vi "102_Lipgap_Full_Algo_new.vi"(0 "Image":T4(plugin-control), 1 "Calibrated Image":T4, 2 "Reference ROI":T5 {"Contours"."Type" items=["No Selection", "Point", "Line", "Rectangle", "Oval", "Polygon", "Freehand Region", "Annulus", "Unused2", "Unused3", "Broken Line", "Freehand Line", "Rotated Rectangle"]}, 3 "Line Options ROI Ref":T9={"Number of Lines"=1, "Type"=enum."First Edge Rake", "Min. Score"=10.0, "Max. Score"=1000.0, "Orientation"=0.0, "Angle Range"=45.0, "Angle Tolerance"=1.0, "Step Size"=3, "Min. SNR (db)"=0.0, "Min. Points (%)"=25.0, "Hough Iterations"=5} {"Min. Points (%)" min=0.0 max=100.0; "Min. SNR (db)" min=0.0; "Max. Score" min=0.0 max=1024.0; "Min. Score" min=0.0 max=1024.0 step=1.0}, 4 "Edge Options ROI Ref":T6={"Edge Polarity"=0, "Kernel Size"=3, "Width"=3, "Minimum Edge Strength"=50.0, "Interpolation Type"=enum."Zero Order", "Data Processing Method"=enum."Average"} {"Edge Polarity" items=["All Edges", "Rising Edges", "Falling Edges"]; "Minimum Edge Strength" format="%.2f"; "Width" step=2; "Kernel Size" step=2}, 5 "Search Direction ROI Ref":u32=3, 6 "Measurement ROI 1":T5 {"Contours"."Type" items=["No Selection", "Point", "Line", "Rectangle", "Oval", "Polygon", "Freehand Region", "Annulus", "Unused2", "Unused3", "Broken Line", "Freehand Line", "Rotated Rectangle"]}, 7 "error in (no error)":errorcluster, 8 "Blob Center":cluster{"Center X":dbl, "Center Y":dbl}, 9 "Search Direction ROI 1":u16(ring)=2 items=["Left To Right", "Right To Left", "Top To Bottom", "Bottom To Top"], 10 "Edge Options ROI 1":T6={"Edge Polarity"=0, "Kernel Size"=3, "Width"=3, "Minimum Edge Strength"=50.0, "Interpolation Type"=enum."Zero Order", "Data Processing Method"=enum."Average"} {"Edge Polarity" items=["All Edges", "Rising Edges", "Falling Edges"]; "Minimum Edge Strength" format="%.2f"; "Width" step=2; "Kernel Size" step=2}, 11 "Measurement ROI 2":T5 {"Contours"."Type" items=["No Selection", "Point", "Line", "Rectangle", "Oval", "Polygon", "Freehand Region", "Annulus", "Unused2", "Unused3", "Broken Line", "Freehand Line", "Rotated Rectangle"]}, 12 "Scan Direction ROI 2":u16(ring) items=["Left To Right", "Right To Left", "Top To Bottom", "Bottom To Top"], 13 "Edge Options ROI 2":T6={"Edge Polarity"=0, "Kernel Size"=3, "Width"=3, "Minimum Edge Strength"=10.0, "Interpolation Type"=enum."Bilinear Fixed", "Data Processing Method"=enum."Average"} {"Edge Polarity" items=["All Edges", "Rising Edges", "Falling Edges"]; "Minimum Edge Strength" format="%.2f"; "Width" step=2; "Kernel Size" step=2}, 14 "Process ROI 2":T8(ring)=enum."Get All Edges", 15 "Step Size ROI 2":u32=5) -> (18 "Overlay Arrow Lines":T1, 20 "Real World Lip Gap 102":sgl, 27 "error IO":errorcluster)   [LabVIEW 2019, in "Algorithm.lvclass"]
uses:
  FrameworkOverrides/Algorithm.lvclass
  <vilib>/vision/NI_Vision_Development_Module.lvlib
  <vilib>/vision/Measure.llb/Edge Polarity.ctl
  <vilib>/vision/Measure.llb/Edge Options.ctl
  <vilib>/vision/Measure.llb/Straight Edge Process.ctl
  <vilib>/vision/Measure.llb/Straight Edge Options.ctl
  <vilib>/vision/Image Controls.llb/IMAQ Image.ctl
panel:
  out "Second Overlay Line":T2
  out "First Overlay Line":T3
  out "Array":i32[](array[numeric])
  out "min value":sgl
  out "max value":sgl
  out "x/y":sgl
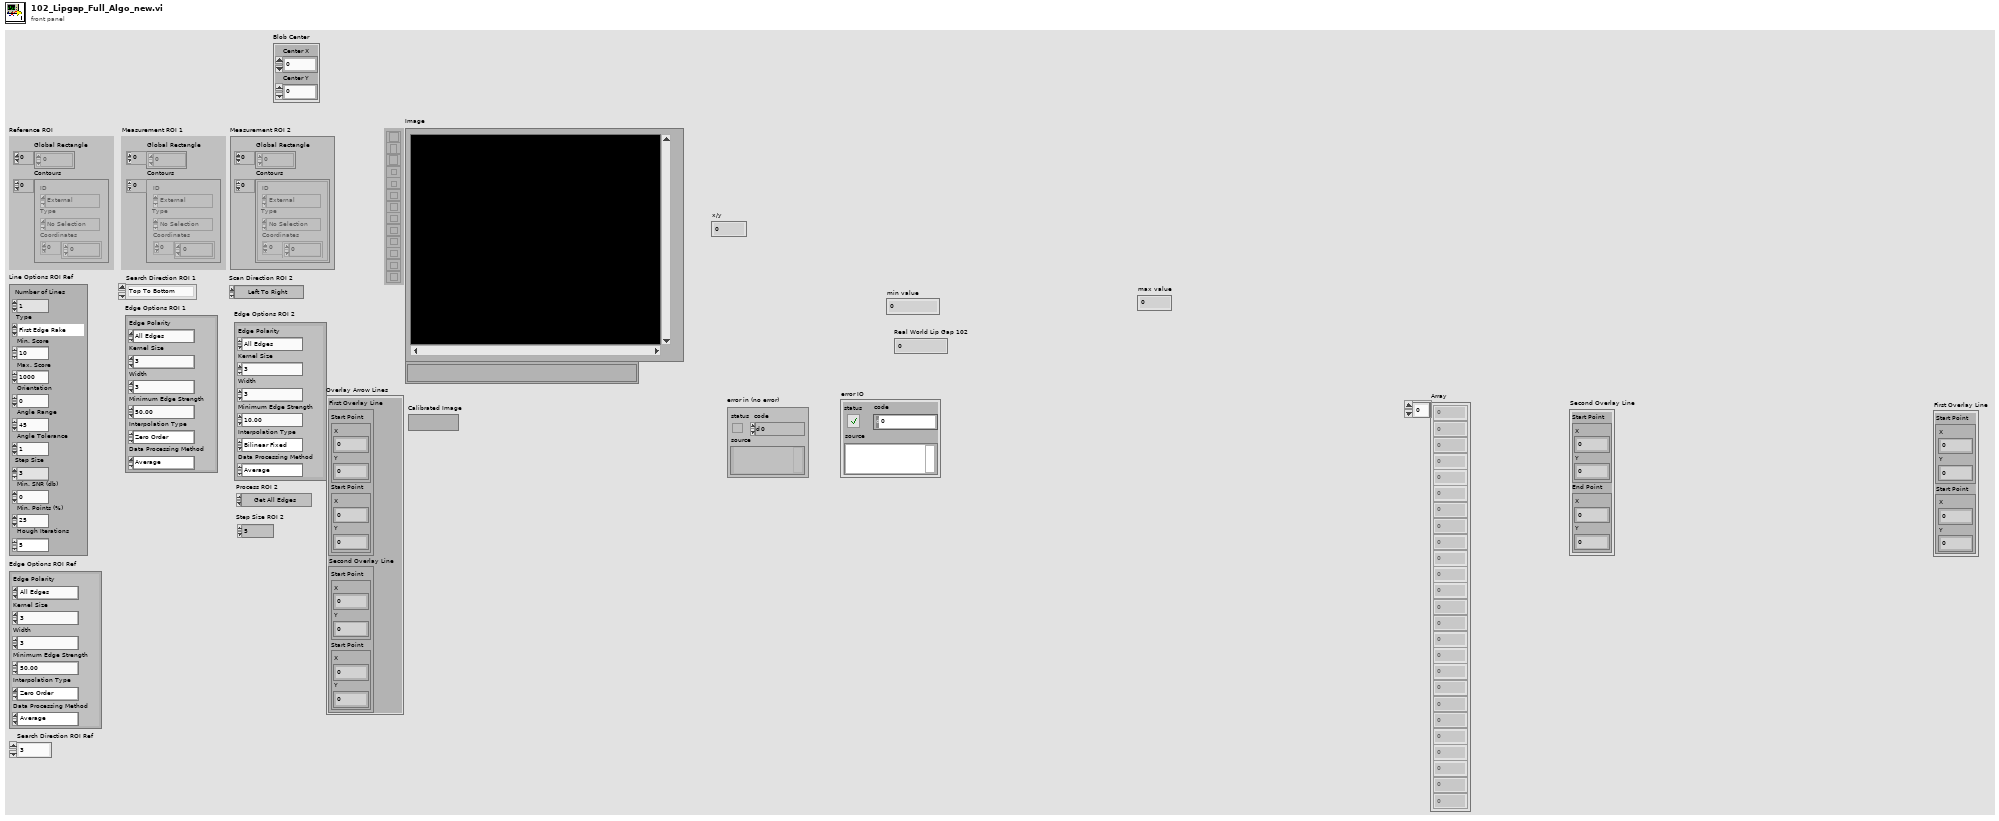
[diagram p1: front panel]
types:
  T1 = cluster{"First Overlay Line ":cluster{"Start Point":cluster{"X":sgl, "Y":sgl}, "Start Point":cluster{"X":sgl, "Y":sgl}}, "Second Overlay Line ":cluster{"Start Point":cluster{"X":sgl, "Y":sgl}, "Start Point":cluster{"X":sgl, "Y":sgl}}}
  T2 = cluster{"Start Point":cluster{"X":sgl, "Y":sgl}, "End Point":cluster{"X":sgl, "Y":sgl}}
  T3 = cluster{"Start Point":cluster{"X":sgl, "Y":sgl}, "Start Point":cluster{"X":sgl, "Y":sgl}}
  T4 = typedef "IMAQ Image.ctl" = refnum<image>
  T5 = typedef "ROI Descriptor" = cluster{"Global Rectangle":i32[], "Contours":cluster{"ID":enum32{"External", "Internal"}, "Type":u32, "Coordinates":i32[]}[]}
  T6 = typedef "Edge Options.ctl" = cluster{"Edge Polarity":T7, "Kernel Size":u32, "Width":u32, "Minimum Edge Strength":sgl, "Interpolation Type":enum32{"Zero Order", "Bilinear", "Quadratic", "Cubic", "Bilinear Fixed"}, "Data Processing Method":enum32{"Average", "Median"}}
  T7 = typedef "Edge Polarity.ctl" = u32
  T8 = enum16{"Get First Edge", "Get First + Last Edge", "Get All Edges", "Get Best Edge"}
  T9 = typedef "Straight Edge Options.ctl" = cluster{"Number of Lines":i32, "Type":T10, "Min. Score":dbl, "Max. Score":dbl, "Orientation":dbl, "Angle Range":dbl, "Angle Tolerance":dbl, "Step Size":u32, "Min. SNR (db)":dbl, "Min. Points (%)":dbl, "Hough Iterations":i32}
  T10 = typedef "Straight Edge Process.ctl" = enum32{"First Edge Rake", "Best Edge Rake", "Hough Edge Rake", "First Edge Projection", "Best Edge Projection"}
  T11 = typedef "IMAQ Rectangle" = cluster{"Left":i32, "Top":i32, "Right":i32, "Bottom":i32, "Rotation":dbl}
  T12 = cluster{"Left":dbl, "Top":dbl, "Right":dbl, "Bottom":dbl, "Angle":dbl}
  T13 = cluster{"Search Direction":u32, "Edge Options":T6, "Show Search Area":bool, "Show Search Lines":bool, "Show Edges Found":bool, "Show Result":bool, "Search Area Color":u32, "Search Lines Color":u32, "Edge Locations Color":u32, "Result Color":u32, "Overlay Group Name":string}
  T14 = cluster{"Point1 (Pixels)":cluster{"X":sgl, "Y":sgl}, "Point2 (Pixels)":cluster{"X":sgl, "Y":sgl}, "Point1 (Real-World)":cluster{"X":sgl, "Y":sgl}, "Point2 (Real-World)":cluster{"X":sgl, "Y":sgl}, "Angle (Pixel)":dbl, "Angle (Real-World)":dbl, "Score":dbl, "Straightness":dbl, "Average SNR (db)":dbl, "Calibration Valid":bool}[]
  T15 = cluster{"Point1 (Pixels)":cluster{"X":sgl, "Y":sgl}, "Point2 (Pixels)":cluster{"X":sgl, "Y":sgl}, "Point1 (Real-World)":cluster{"X":sgl, "Y":sgl}, "Point2 (Real-World)":cluster{"X":sgl, "Y":sgl}, "Angle (Pixel)":dbl, "Angle (Real-World)":dbl, "Score":dbl, "Straightness":dbl, "Average SNR (db)":dbl, "Calibration Valid":bool}
  T16 = typedef "IMAQ Line" = cluster{"Start X":i32, "Start Y":i32, "End X":i32, "End Y":i32}
  T17 = typedef "Search Line.ctl" = cluster{"Start Point":cluster{"X":sgl, "Y":sgl}, "End Point":cluster{"X":sgl, "Y":sgl}, "Edge Info":T18[], "Edge Map":dbl[], "Calibration Valid":bool}
  T18 = typedef "Edge New.ctl" = cluster{"Location (Pixel)":cluster{"X":sgl, "Y":sgl}, "Location (Real-World)":cluster{"X":sgl, "Y":sgl}, "Distance (Pixel)":dbl, "Distance (Real-World)":dbl, "Strength":dbl, "Noise":dbl, "Rising?":bool}
  T19 = cluster{"Start Point":cluster{"X":sgl, "Y":sgl}, "Location (Pixel)":cluster{"X":sgl, "Y":sgl}}
  T20 = cluster{"Location (Pixel)":cluster{"X":sgl, "Y":sgl}, "End Point":cluster{"X":sgl, "Y":sgl}}
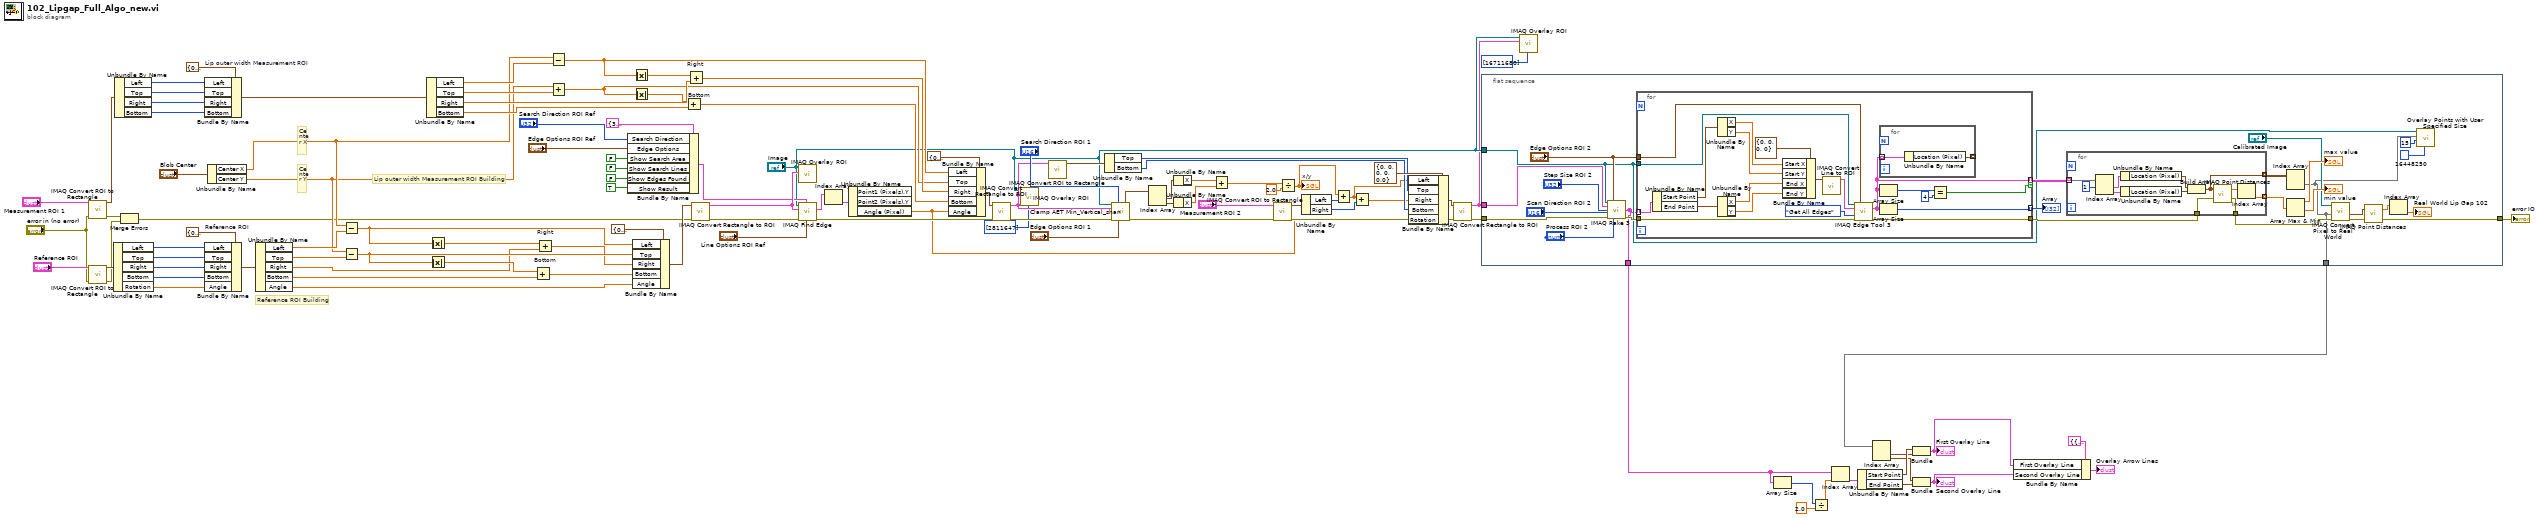
[diagram p0: block diagram]
diagram:
  # "Lip outer width Measurement ROI Building"
  # "Reference ROI Building"
  # "Center Y"
  # "Center X"
  n1 = call "IMAQ Convert ROI to Rectangle"("error in (no error)"="error in (no error)", "ROI Descriptor"="Measurement ROI 1") -> ("error out"=w58:errorcluster, "Rectangle"=w69:T11)  [unwired: 7 in]
  n2 = call "IMAQ Convert ROI to Rectangle"("error in (no error)"="error in (no error)", "ROI Descriptor"="Reference ROI") -> ("error out"=w57:errorcluster, "Rectangle"=w64:T11)  [unwired: 7 in]
  n3 = Unbundle By Name(w64) -> ("Left"=w63:i32, "Top"=w62:i32, "Right"=w61:i32, "Bottom"=w60:i32, "Rotation"=w59:dbl)
  n4 = Unbundle By Name(w69) -> ("Left"=w68:i32, "Top"=w67:i32, "Right"=w66:i32, "Bottom"=w65:i32)
  n5 = Merge Errors(w58, w57) -> (w56:errorcluster)
  n6 = Bundle By Name "Lip outer width Measurement ROI"(cluster=T12 {"Left"=0.0, "Top"=0.0, "Right"=0.0, "Bottom"=0.0, "Angle"=0.0} ("input cluster"), "Left"=w68, "Top"=w67, "Right"=w66, "Bottom"=w65) -> (w77:T12)
  n7 = Bundle By Name "Reference ROI"(cluster=T12 {"Left"=0.0, "Top"=0.0, "Right"=0.0, "Bottom"=0.0, "Angle"=0.0} ("input cluster"), "Left"=w63, "Top"=w62, "Right"=w61, "Bottom"=w60, "Angle"=w59) -> (w76:T12)
  n8 = Unbundle By Name("Blob Center") -> ("Center X"=w71:dbl, "Center Y"=w70:dbl)
  n9 = Unbundle By Name(w76) -> ("Left"=w102:dbl, "Top"=w101:dbl, "Right"=w100:dbl, "Bottom"=w99:dbl, "Angle"=w98:dbl)
  n10 = Subtract(x=w71, y=w102) -> (x-y=w106:dbl)
  n11 = Subtract(x=w70, y=w101) -> (x-y=w105:dbl)
  n12 = Unbundle By Name(w77) -> ("Left"=w85:dbl, "Top"=w84:dbl, "Right"=w83:dbl, "Bottom"=w82:dbl)
  n13 = Absolute Value(x=w106) -> (abs(x)=w109:dbl)
  n14 = Absolute Value(x=w105) -> (abs(x)=w108:dbl)
  n15 = Add "Bottom"(x=w108, y=w99) -> (x+y=w103:dbl)
  n16 = Add "Right"(x=w109, y=w100) -> (x+y=w104:dbl)
  n17 = Subtract(x=w71, y=w85) -> (x-y=w88:dbl)
  n18 = Add(x=w70, y=w84) -> (x+y=w80:dbl)
  n19 = Bundle By Name(cluster=T13 {"Search Direction"=3, "Edge Options"={"Edge Polarity"=0, "Kernel Size"=3, "Width"=3, "Minimum Edge Strength"=50.0, "Interpolation Type"=enum."Zero Order", "Data Processing Method"=enum."Average"}, "Show Search Area"=FALSE, "Show Search Lines"=FALSE, "Show Edges Found"=FALSE, "Show Result"=TRUE, "Search Area Color"=65280, "Search Lines Color"=255, "Edge Locations Color"=16776960, "Result Color"=16711680, "Overlay Group Name"=""} ("Options"), "Search Direction"="Search Direction ROI Ref", "Edge Options"="Edge Options ROI Ref", "Show Search Area"=FALSE, "Show Search Lines"=FALSE, "Show Edges Found"=FALSE, "Show Result"=TRUE) -> (w51:T13)
  n20 = Absolute Value(x=w88) -> (abs(x)=w90:dbl)
  n21 = Absolute Value(x=w80) -> (abs(x)=w81:dbl)
  n22 = Bundle By Name(cluster=T12 {"Left"=0.0, "Top"=0.0, "Right"=0.0, "Bottom"=0.0, "Angle"=0.0} ("input cluster"), "Left"=w106, "Top"=w105, "Right"=w104, "Bottom"=w103, "Angle"=w98) -> (w93:T12)
  n23 = Add "Bottom"(x=w81, y=w82) -> (x+y=w86:dbl)
  n24 = Add "Right"(x=w90, y=w83) -> (x+y=w87:dbl)
  n25 = call "IMAQ Convert Rectangle to ROI"("error in (no error)"=w56, "Rectangle"=w93) -> ("error out"=w97:errorcluster, "ROI Descriptor"=w91:T5)  [unwired: 7 in]
  n26 = call "IMAQ Overlay ROI"("ROI Descriptor"=w91, "Image"="Image") -> ()  [unwired: 8 in, 2 out]
  n27 = call "IMAQ Find Edge"("Line Fit Options"="Line Options ROI Ref", "Options"=w51, "error in (no error)"=w97, "ROI Descriptor"=w91, "Image"="Image") -> ("error out"=w55:errorcluster, "Straight Edges"=w95:T14)  [unwired: 3 in, 2 out]
  n28 = Index Array(array=w95) -> (element=w94:T15)  [unwired: 1 in]
  n29 = Unbundle By Name(w94) -> ("Angle (Pixel)"=w15:dbl)  [unwired: 2 out]
  n30 = Bundle By Name(cluster=T12 {"Left"=0.0, "Top"=0.0, "Right"=0.0, "Bottom"=0.0, "Angle"=0.0} ("input cluster"), "Left"=w88, "Top"=w80, "Right"=w87, "Bottom"=w86, "Angle"=w15) -> (w79:T12)
  n31 = call "IMAQ Convert Rectangle to ROI"("error in (no error)"=w55, "Rectangle"=w79) -> ("error out"=w75:errorcluster, "ROI Descriptor"=w36:T5)  [unwired: 7 in]
  n32 = call "IMAQ Overlay ROI"("Colors (Green)"=u32[] [2811647], "ROI Descriptor"=w36, "Image"="Image") -> ()  [unwired: 7 in, 2 out]
  n33 = call "IMAQ Convert ROI to Rectangle"("ROI Descriptor"=w36) -> ("Rectangle"=w35:T11)  [unwired: 8 in, 1 out]
  n34 = Unbundle By Name(w35) -> ("Top"=w33:i32, "Bottom"=w32:i32)
  n35 = call "Clamp AET Min_Vertical_shan.vi"("Image"="Image", "Scanning axis"="Search Direction ROI 1", "ROI Descriptor"=w36, "error in (no error)"=w75, "Edge Options"="Edge Options ROI 1") -> ("Edge Coordinates"=w44:cluster{"X":sgl, "Y":sgl}[], "error out"=w20:errorcluster)  [unwired: 4 in, 5 out]
  n36 = Index Array(array=w44) -> (element #1=w43:cluster{"X":sgl, "Y":sgl}, element #2=w42:cluster{"X":sgl, "Y":sgl})  [unwired: 2 in]
  n37 = Unbundle By Name(w43) -> ("X"=w41:sgl)
  n38 = Unbundle By Name(w42) -> ("X"=w40:sgl)
  n39 = Add(x=w41, y=w40) -> (x+y=w39:sgl)
  n40 = call "IMAQ Convert ROI to Rectangle"("error in (no error)"=w20, "ROI Descriptor"="Measurement ROI 2") -> ("error out"=w19:errorcluster, "Rectangle"=w24:T11)  [unwired: 7 in]
  n41 = Divide(x=w39, y=sgl 2.0) -> (x/y=w37:sgl)
  "x/y" <- w37
  n42 = Unbundle By Name(w24) -> ("Left"=w22:i32, "Right"=w21:i32)
  n43 = Add(x=w37, y=w22) -> (x+y=w31:sgl)
  n44 = Add(x=w31, y=w21) -> (x+y=w30:sgl)
  n45 = Bundle By Name(cluster=T11 {"Left"=0, "Top"=0, "Right"=0, "Bottom"=0, "Rotation"=0.0} ("Rectangle"), "Left"=w31, "Top"=w33, "Right"=w30, "Bottom"=w32, "Rotation"=w15) -> (w29:T11)
  n46 = call "IMAQ Convert Rectangle to ROI"("error in (no error)"=w19, "Rectangle"=w29) -> ("error out"=w25:errorcluster, "ROI Descriptor"=w26:T5)  [unwired: 7 in]
  n47 = flat-sequence {
    tunnel: "Image" -> [w112]
    tunnel: w26 -> [w120]
    tunnel: w25 -> [w119]
    tunnel: [w117] -> w17
    tunnel: [w111] -> w3
    tunnel: [w110] -> w2
    frame #0 {
      n48 = call "IMAQ Rake 3"("Image"=w112, "Edge Options"="Edge Options ROI 2", "ROI Descriptor"=w120, "Step Size"="Step Size ROI 2", "Scan Direction"="Scan Direction ROI 2", "error in (no error)"=w119, "Process"="Process ROI 2") -> ("Search Lines"=w110:T17[], "error out"=w131:errorcluster)  [unwired: 5 in, 2 out]
      n49 = for {
        tunnel: w110 -> [w166] mode=indexing
        tunnel: w112 -> [w156]
        tunnel: "Edge Options ROI 2" -> [w157]
        tunnel: w131 -> [w155]
        tunnel: [w154] -> w114
        tunnel: [w151] -> w130 mode=indexing
        tunnel: [w150] -> w129 mode=indexing if=w147
        n50 = Unbundle By Name(w166) -> ("Start Point"=w153:cluster{"X":sgl, "Y":sgl}, "End Point"=w152:cluster{"X":sgl, "Y":sgl})
        n51 = Unbundle By Name(w153) -> ("X"=w164:sgl, "Y"=w163:sgl)
        n52 = Unbundle By Name(w152) -> ("X"=w162:sgl, "Y"=w161:sgl)
        n53 = Bundle By Name(cluster=T16 {"Start X"=0, "Start Y"=0, "End X"=0, "End Y"=0} ("Line"), "Start X"=w164, "Start Y"=w163, "End X"=w162, "End Y"=w161) -> (w160:T16)
        n54 = call "IMAQ Convert Line to ROI"("Line"=w160) -> ("ROI Descriptor"=w159:T5)  [unwired: 8 in, 1 out]
        n55 = call "IMAQ Edge Tool 3"("Image"=w156, "Edge Options"=w157, "ROI Descriptor"=w159, "Process"=T8."Get All Edges", "error in (no error)"=w155) -> ("Edge Information"=w150:T18[], "error out"=w154:errorcluster)  [unwired: 6 in, 3 out]
        n56 = for {
          tunnel: w150 -> [w168] mode=indexing
          tunnel: [w167] -> _ mode=indexing
          n57 = Unbundle By Name(w168) -> ("Location (Pixel)"=w167:cluster{"X":sgl, "Y":sgl})
        }
        n58 = Array Size(array=w150) -> (size(s)=w149:i32)
        n59 = Array Size(array=w150) -> (size(s)=w151:i32)
        n60 = Equal?(x=w149, y=4) -> (x = y?=w147:bool)
      }
      "Array" <- w130
      n61 = for {
        tunnel: w129 -> [w146] mode=indexing
        tunnel: [w139] -> w128 mode=indexing
        tunnel: [w138] -> w125 mode=indexing
        tunnel: w114 -> [w137]
        tunnel: [w136] -> w113
        n62 = Index Array(array=w146, index #1=1 ("index")) -> (element #1=w144:T18, element #2=w143:T18)  [unwired: 1 in]
        n63 = Unbundle By Name(w144) -> ("Location (Pixel)"=w142:cluster{"X":sgl, "Y":sgl})
        n64 = Unbundle By Name(w143) -> ("Location (Pixel)"=w141:cluster{"X":sgl, "Y":sgl})
        n65 = Build Array(w142, w141) -> (w138:cluster{"X":sgl, "Y":sgl}[])
        n66 = call "IMAQ Point Distances"("Points"=w138, "error in (no error)"=w137) -> ("Distances"=w140:sgl[], "error out"=w136:errorcluster)  [unwired: 3 in]
        n67 = Index Array(array=w140) -> (element=w139:sgl)  [unwired: 1 in]
      }
      n68 = Index Array(array=w125) -> (element=w111:cluster{"X":sgl, "Y":sgl}[])  [unwired: 2 in]
      n69 = Array Max & Min(array=w128) -> (max value=→"max value":sgl, min value=→"min value":sgl)  [unwired: 2 out]
      n70 = call "IMAQ Convert Pixel to Real World"("error in (no error)"=w113, "Array of Pixel Coordinates"=w111, "Calibrated Image"="Calibrated Image") -> ("error out"=w123:errorcluster, "Array of Real World Coordinates"=w124:cluster{"X":sgl, "Y":sgl}[])  [unwired: 3 in, 4 out]
      n71 = call "IMAQ Point Distances"("Points"=w124, "error in (no error)"=w123) -> ("Distances"=w122:sgl[], "error out"=w117:errorcluster)  [unwired: 3 in]
      n72 = Index Array(array=w122) -> (element=→"Real World Lip Gap 102":sgl)  [unwired: 1 in]
      n73 = call "Overlay Points with User Specified Size.vi"("Color"=u32 16448250, "Point Diameter (5)"=u32 15, "Points"=w111, "Image In"=w112) -> ()  [unwired: 6 in, 2 out]
    }
  }
  n74 = call "IMAQ Overlay ROI"("Colors (Green)"=u32[] [16711680], "ROI Descriptor"=w26, "Image"="Image") -> ()  [unwired: 7 in, 2 out]
  n75 = Array Size(array=w2) -> (size(s)=w5:i32)
  n76 = Divide(x=w5, y=2.0) -> (x/y=w4:dbl)
  n77 = Index Array(array=w2, index=w4) -> (element=w14:T17)
  n78 = Unbundle By Name(w14) -> ("Start Point"=w13:cluster{"X":sgl, "Y":sgl}, "End Point"=w10:cluster{"X":sgl, "Y":sgl})
  n79 = Index Array(array=w3) -> (element #1=w12:cluster{"X":sgl, "Y":sgl}, element #2=w11:cluster{"X":sgl, "Y":sgl})  [unwired: 2 in]
  n80 = Bundle("Start Point"=w13, "Location (Pixel)"=w12) -> (w8:T19)  [unwired: 1 in]
  "First Overlay Line" <- w8
  n81 = Bundle("Location (Pixel)"=w11, "End Point"=w10) -> (w7:T20)  [unwired: 1 in]
  "Second Overlay Line" <- w7
  n82 = Bundle By Name(cluster=T1 {"First Overlay Line "={"Start Point"={"X"=0.0, "Y"=0.0}, "Start Point"={"X"=0.0, "Y"=0.0}}, "Second Overlay Line "={"Start Point"={"X"=0.0, "Y"=0.0}, "Start Point"={"X"=0.0, "Y"=0.0}}}, "First Overlay Line"=w8, "Second Overlay Line"=w7) -> (→"Overlay Arrow Lines":T1)
  "error IO" <- w17
